vi "Printer Error Handler.vi"(8 "entrée d'erreur (pas d'erreur)":errorcluster, 11 "État en entrée":T1) -> (0 "sortie d'erreur":errorcluster, 3 "État suivant":T1)   [LabVIEW 2009]
doc: "Utilisez ce modèle pour construire un VI à utiliser en tant que sous-VI."
uses:
  Print Processing States.ctl
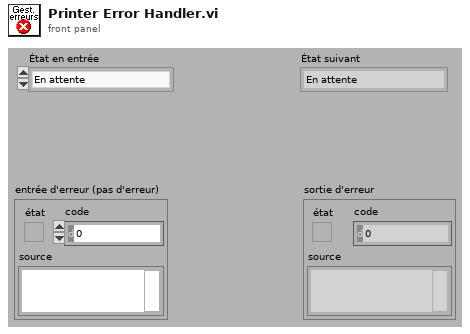
[diagram p1: front panel]
types:
  T1 = typedef "Print Processing States.ctl" = enum16{"En attente", "Initialisation de la configuration", "Configuration", "Initialisation de l'impression", "Impression", "Arrêt"}
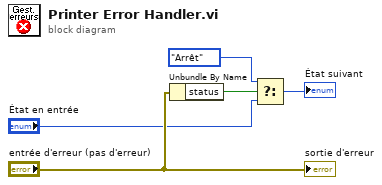
[diagram p0: block diagram]
diagram:
  n1 = Unbundle By Name ("Désassembler par nom")("entrée d'erreur (pas d'erreur)") -> ("status"=w1:bool)
  n2 = Select ("Sélectionner")(t=Print_Processing_States."Arrêt", s=w1, f="État en entrée") -> (s? t:f=→"État suivant":T1)
  "sortie d'erreur" <- "entrée d'erreur (pas d'erreur)"
